vi "Get Plugin Metadata.vi"(8 "error in (no error)":errorcluster, 10 "Plugin Types Tree":refnum<vi>, 11 "CIF_UI in":refnum<class "CIF_Manager_UI.lvclass">) -> (0 "error out":errorcluster, 2 "plugin_metadata":T1)   [LabVIEW 2021, in "CIF_Manager_UI.lvclass"]
uses:
  CIF_Manager_UI.lvclass
  <vilib>/CIF Foundation/CIF Core/CIFPluginManager/gRPC/CIF_Manager_client/RPC Messages/cif_management_common_PluginMetadata.ctl
  CIF_Manager_UI.lvclass/CIF_Manager_UI.ctl
  <vilib>/CIF Foundation/CIF Core/CIFPluginManager/gRPC/CIF_Manager_client/CIF_Manager_client.lvlib
  <vilib>/CIF Foundation/CIF Core/CIFCore/Common/CIFCoreCommon.lvlib
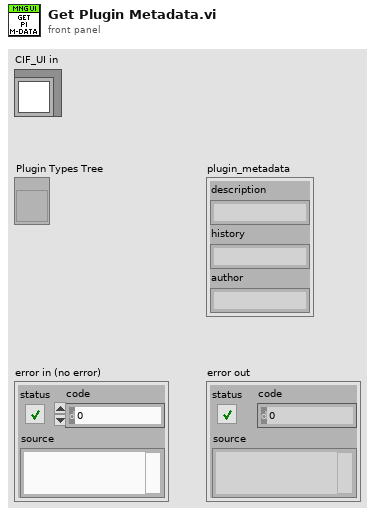
[diagram p1: front panel]
types:
  T1 = typedef "CIF_Manager_client.lvlib/cif_management_common_PluginMetadata.ctl" = cluster{"description":string, "history":string, "author":string}
  T2 = typedef "CIF_Manager_client.lvlib/cif_manager_PluginType.ctl" = cluster{"plugin_type":string, "plugin_version":T3, "plugin_metadata":T1, "relative_path":string[]}
  T3 = typedef "CIF_Manager_client.lvlib/cif_common_ShortVersion.ctl" = cluster{"major":u32, "minor":u32, "fix":u32}
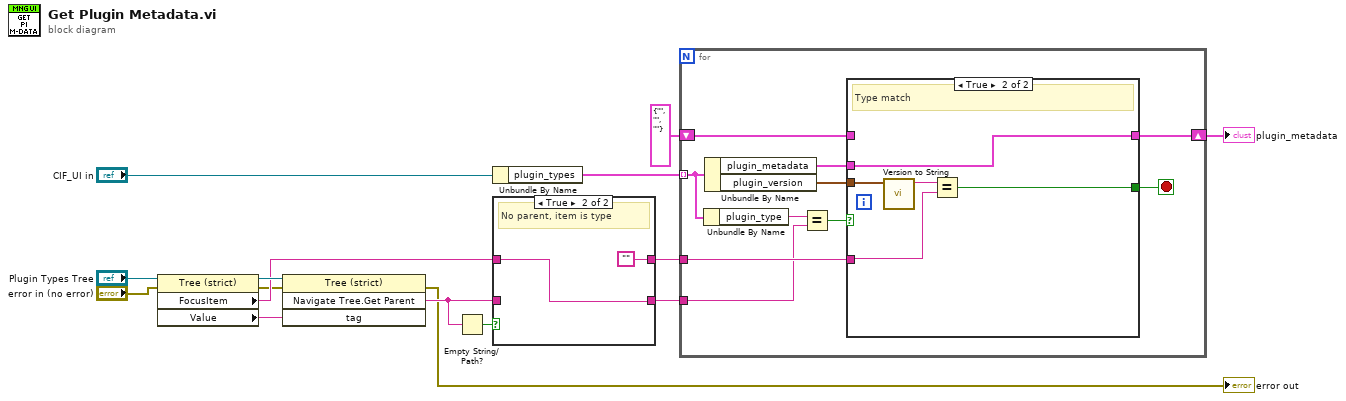
[diagram p0: block diagram]
diagram:
  n1 = property class="Tree (strict)"(reference="Plugin Types Tree", error in="error in (no error)") -> (error out=w9:errorcluster, "FocusItem"=w10:string, "Value"=w14:string)  [unwired: 1 out]
  n2 = invoke class="Tree (strict)" method="Navigate Tree.Get Parent"(reference="Plugin Types Tree", error in=w9, "tag"=w14) -> (error out=→"error out":errorcluster, "Navigate Tree:Get Parent"=w11:string)  [unwired: 1 in, 2 out]
  n3 = Empty String/Path?(string/path=w11) -> (empty?=w12:bool)
  n4 = Unbundle By Name("CIF_UI in") -> ("plugin_types"=w4:T2[])
  n5 = case shown="True" w12 {
    tunnel: w11 -> [w15 _]
    tunnel: w10 -> [w16 w18]
    tunnel: [w16 ""] -> w7
    tunnel: [w15 w18] -> w8
    frame False {
      # "Parent is type, item is version"
    }
    frame True {
      # "No parent, item is type"
    }
  }
  n6 = for {
    tunnel: w8 -> [w27]
    tunnel: w7 -> [w28]
    tunnel: w4 -> [w24] mode=indexing
    shift-right: [w21] -> w1
    shift-left: T1 {"description"="", "history"="", "author"=""} ("plugin_metadata") -> [w20]
    stop <- w19 stop-if-true
    n7 = Unbundle By Name(w24) -> ("plugin_type"=w26:string)
    n8 = Unbundle By Name(w24) -> ("plugin_metadata"=w22:T1, "plugin_version"=w23:T3)
    n9 = Equal?(x=w26, y=w27) -> (x = y?=w25:bool)
    n10 = case shown="True" w25 {
      tunnel: w28 -> [_ w33]
      tunnel: w23 -> [_ w34]
      tunnel: w22 -> [_ w31]
      tunnel: [w29 w31] -> w21
      tunnel: [_ w30] -> w19
      tunnel: w20 -> [w29 _]
      frame False {
        # "Wrong Type"
      }
      frame True {
        # "Type match"
        n11 = call <vilib>:"Version to String.vi"("Version"=w34) -> ("Version String"=w32:string)  [unwired: 10 in]
        n12 = Equal?(x=w32, y=w33) -> (x = y?=w30:bool)
      }
    }
  }
  "plugin_metadata" <- w1
